vi "PL Close.vi"(8 "error in":errorcluster, 9 "Notifiers":T1, 10 "User Event":refnum<user-event>, 11 "Event Registration Refnum in":refnum<event-registration>) -> (0 "error out":errorcluster)   [LabVIEW 2014]
doc: "Closes references to main application resources (notifiers, user events etc.)"
uses:
  User Event - EHL Stop/User Event - EHL Stop.lvlib
  Notifiers/Notifiers.lvlib
  Notifiers/Notifiers.ctl
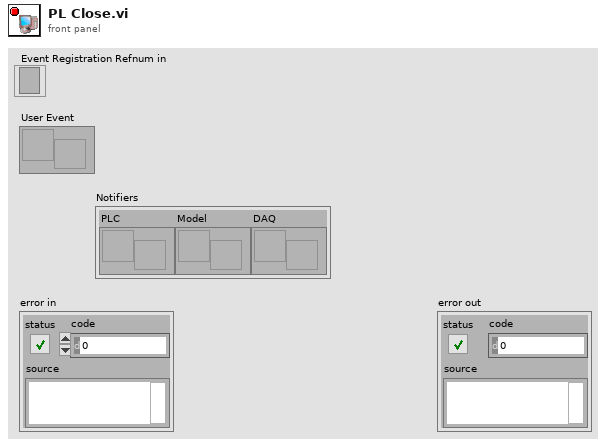
[diagram p1: front panel]
types:
  T1 = typedef "Notifiers.lvlib/Notifiers.ctl" = cluster{"PLC":refnum<notifier>, "Model":refnum<notifier>, "DAQ":refnum<notifier>}
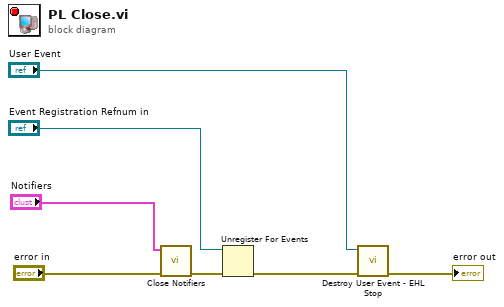
[diagram p0: block diagram]
diagram:
  n1 = call "Close Notifiers.vi"("error in"="error in", "Notifiers"="Notifiers") -> ("error out"=w6:errorcluster)  [unwired: 9 in]
  n2 = Unregister For Events(event registration refnum="Event Registration Refnum in", error in=w6) -> (error out=w7:errorcluster)
  n3 = call "Destroy User Event - EHL Stop.vi"("error in"=w7, "User Event"="User Event") -> ("error out"=→"error out":errorcluster)  [unwired: 9 in]
